vi "Read an entire module using API.vi"() -> ()   [LabVIEW 2025]
uses:
  <resource>/objmgr/cRIO.rc
panel:
  out "Data":dbl[](array[numeric])
  in  "stop":bool
  out "error out":errorcluster
  out "All Variables[]":refnum<k21>[](array[refnum])
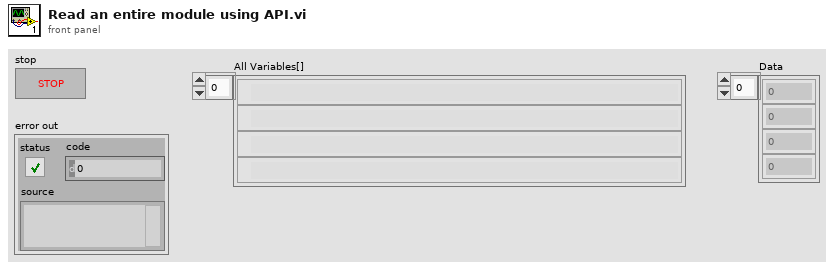
[diagram p1: front panel]
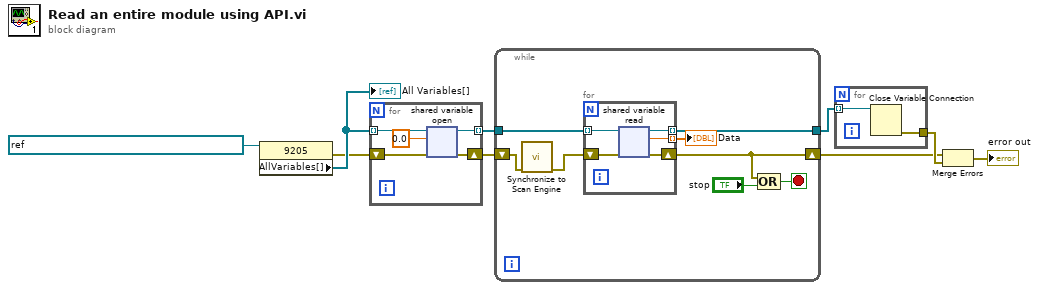
[diagram p0: block diagram]
diagram:
  n1 = property class="9205"(reference=refnum<k21> "ni.var.io://ni-crio-9045-01ceedf1/Mod4" ("9205 Refnum")) -> (error out=w6:errorcluster, "AllVariables[]"=w8:refnum<k21>[])  [unwired: 1 in, 1 out]
  "All Variables[]" <- w8
  n2 = for {
    tunnel: w8 -> [w14] mode=indexing
    tunnel: [w12] -> w7 mode=indexing
    shift-right: [w11] -> w5
    shift-left: w6 -> [w10]
    n3 = shared-variable-open(w14, w10, 0.0) -> (w12:refnum<k21>, w11:errorcluster)  [unwired: 1 in]
  }
  n4 = while {
    tunnel: w7 -> [w22]
    shift-right: [w17] -> w2
    shift-left: w5 -> [w21]
    tunnel: [w15] -> w4
    stop <- w16 stop-if-true
    n5 = call <vilib>:"Synchronize to Scan Engine.vi"("error in (no error)"=w21) -> ("error out"=w20:errorcluster)  [unwired: 9 in, 1 out]
    n6 = for {
      tunnel: w22 -> [w27] mode=indexing
      tunnel: [w25] -> w19 mode=indexing
      shift-right: [w24] -> w17
      shift-left: w20 -> [w26]
      tunnel: [w23] -> w15 mode=indexing
      n7 = shared-variable-read(w27, w26) -> (w23:refnum<k21>, w24:errorcluster, w25:dbl)  [unwired: 1 out]
    }
    "Data" <- w19
    n8 = Compound Arithmetic op=OR(w17, "stop") -> (w16:bool)
  }
  n9 = for {
    tunnel: w4 -> [w29] mode=indexing
    tunnel: [w28] -> w3
    n10 = Close Variable Connection(11:w29) -> (0:w28:errorcluster)  [unwired: 1 in]
  }
  n11 = Merge Errors(w2, w3) -> (→"error out":errorcluster)
